vi "Main.vi"   [LabVIEW 2020]
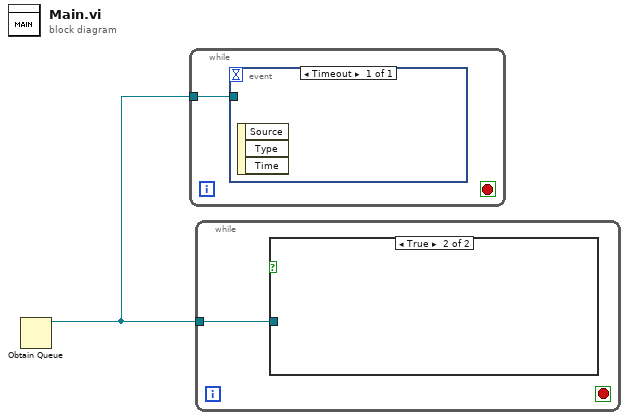
[diagram p0: block diagram]
diagram:
  n1 = Obtain Queue() -> (queue out=w1:refnum<queue>)  [unwired: 5 in, 2 out]
  n2 = while {
    tunnel: w1 -> [w2]
    stop <- _ stop-if-true
    n3 = event shown="[0] Timeout" {
      selector: _ -> [_]
      dyn-events: _ -> [_]
      timeout: _ -> [_]
      tunnel: w2 -> [_]
      event Timeout {
        n4 = event-data() -> ()  [unwired: 1 in, 3 out]
      }
    }
  }
  n5 = while {
    tunnel: w1 -> [w3]
    stop <- _ stop-if-true
    n6 = case shown="True" {
      selector: _ -> [_ _]
      tunnel: w3 -> [_ _]
      frame False {
      }
      frame True {
      }
    }
  }
